vi "Ko.vi"(8 "Model":T3=enum."Gallas", 9 "Thermo and Transport Properties":T1, 10 "SJ Geometry":T2, 11 "omega":dbl=0.001) -> (2 "Ko":dbl=2.000052200153926)   [LabVIEW 2012]
uses:
  Model.ctl
  Utilities/fluid_properties/fluid_properties.ctl
  <vilib>/Analysis/2dsp.llb/Integral Method.ctl
  <vilib>/Analysis/8numeric.llb/1D Numeric Integration.vi
  <vilib>/Analysis/1siggen.llb/Ramp Pattern by Samples.vi
  <vilib>/Analysis/1siggen.llb/Ramp Pattern by Delta.vi
  <vilib>/Analysis/NI_AALBase.lvlib
  <vilib>/Analysis/NI_AALPro.lvlib
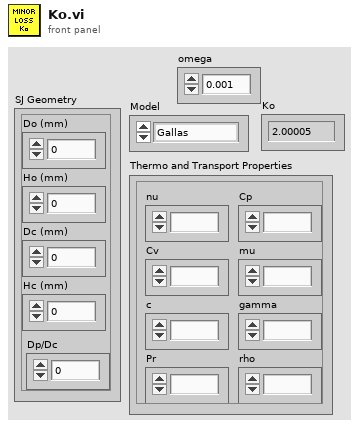
[diagram p1: front panel]
types:
  T1 = typedef "fluid_properties.ctl" = cluster{"nu":dbl, "c":dbl, "Pr":dbl, "Cp":dbl, "Cv":dbl, "gamma":dbl, "mu":dbl, "rho":dbl}
  T2 = cluster{"Do (mm)":dbl, "Ho (mm)":dbl, "Dc (mm)":dbl, "Hc (mm)":dbl, "Dp/Dc":dbl}
  T3 = typedef "Model.ctl" = enum16{"Martin", "Tang", "Gallas", "Persoon"}
  T4 = typedef "NI_AALPro.lvlib/Integral Method.ctl" = i32
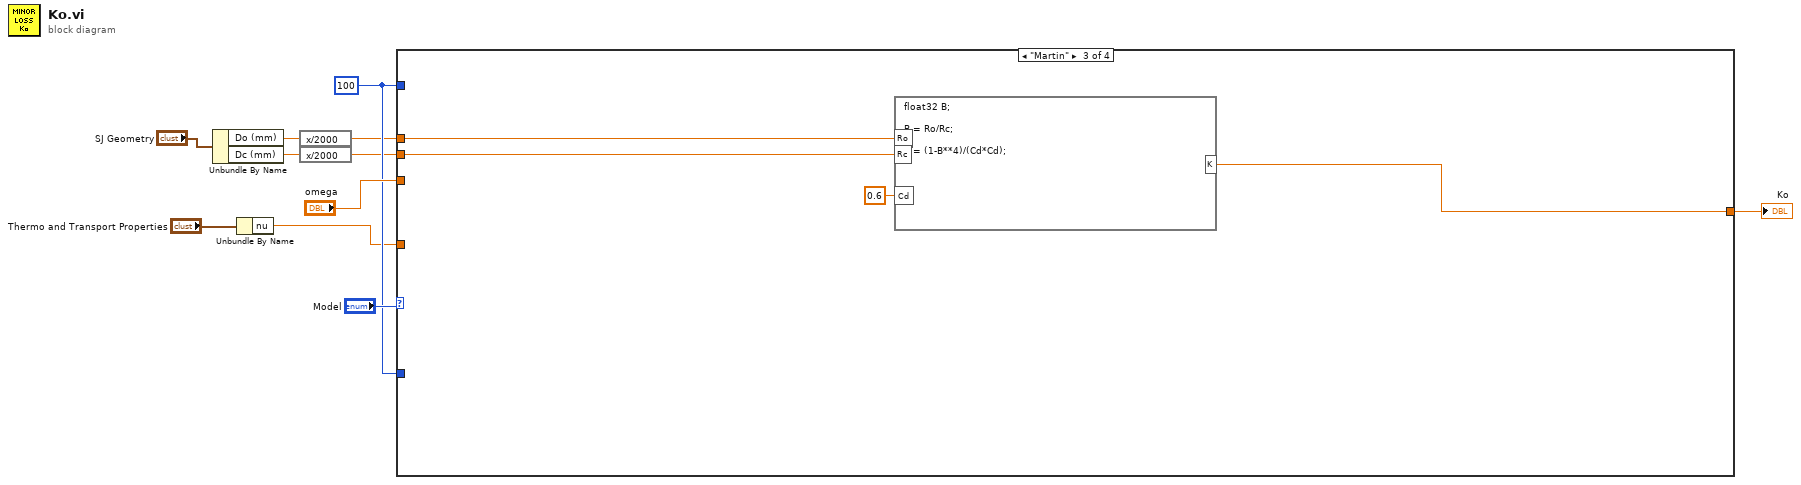
[diagram p0: block diagram]
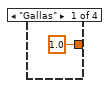
[diagram p2: hidden frame]
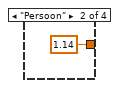
[diagram p3: hidden frame]
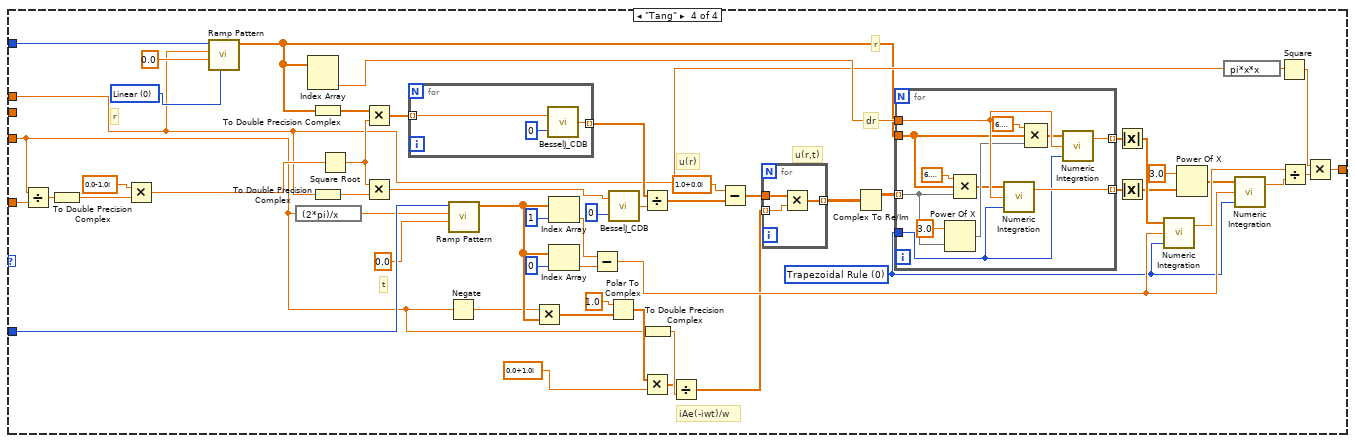
[diagram p4: hidden frame]
diagram:
  w9 = 100 ("n radial pts")
  n1 = Unbundle By Name("SJ Geometry") -> ("Do (mm)"=w7:dbl, "Dc (mm)"=w2:dbl)
  n2 = Unbundle By Name("Thermo and Transport Properties") -> ("nu"=w4:dbl)
  n3 = expression code="x/2000"(w7) -> (w6:dbl)
  n4 = expression code="x/2000"(w2) -> (w1:dbl)
  n5 = case shown="\"Martin\"" "Model" {
    tunnel: [1.0 1.14 w14 w72] -> w3
    tunnel: w4 -> [_ _ _ w57]
    tunnel: w9 -> [_ _ _ w36]
    tunnel: w9 -> [_ _ _ w32]
    tunnel: "omega" -> [_ _ _ w29]
    tunnel: w6 -> [_ _ w17 w27]
    tunnel: w1 -> [_ _ w16 _]
    frame "Gallas" {
    }
    frame "Persoon" {
    }
    frame "Martin" {
      n6 = formula code="float32 B;\n\nB = Ro/Rc;\n\nK = (1-B**4)/(Cd*Cd);"("Ro"=w17, "Rc"=w16, "Cd"=0.6 ("input variable")) -> ("K"=w14:dbl)
    }
    frame "Tang" {
      w23 = T4 0 items=["Trapezoidal Rule", "Simpson's Rule", "Simpson's 3/8 Rule", "Bode Rule"] ("integration method")
      w33 = u16 0 items=["Linear", "Logarithmic"] ("type")
      # "r"
      # "r"
      # "dr"
      # "u(r)"
      # "u(r,t)"
      # "t"
      # "iAe(-iwt)/w"
      n7 = Divide(x=w29, y=w57) -> (x/y=w58:dbl)
      n8 = To Double Precision Complex(1:w58) -> (0:w59:cdb)
      n9 = Multiply(x=cdb 0.0-1.0i, y=w59) -> (x*y=w60:cdb)
      n10 = call-poly <vilib>:"Ramp Pattern.vi"("type"=w33, "start"=0.0, "end"=w27, "samples"=w32) -> ("Ramp Pattern"=w24:dbl[])  [unwired: 6 in, 1 out]
      n11 = expression code="(2*pi)/x"(w29) -> (w28:dbl)
      n12 = Index Array(array=w24) -> (element #2=w31:dbl)  [unwired: 2 in, 1 out]
      n13 = To Double Precision Complex(1:w24) -> (0:w25:cdb[])
      n14 = To Double Precision Complex(1:w27) -> (0:w30:cdb)
      n15 = Square Root(x=w60) -> (sqrt(x)=w62:cdb)
      n16 = Multiply(x=w25, y=w62) -> (x*y=w61:cdb[])
      n17 = Multiply(x=w62, y=w30) -> (x*y=w20:cdb)
      n18 = for {
        tunnel: w61 -> [w75] mode=indexing
        tunnel: [w73] -> w63 mode=indexing
        n19 = call "BesselJ_CDB.vi"("n"=0, "a+bi"=w75) -> ("Jn(a+bi)"=w73:cdb)
      }
      n20 = Negate(x=w29) -> (-x=w43:dbl)
      n21 = call-poly <vilib>:"Ramp Pattern.vi"("start"=0.0, "end"=w28, "samples"=w36) -> ("Ramp Pattern"=w69:dbl[])  [unwired: 7 in, 1 out]
      n22 = Multiply(x=w43, y=w69) -> (x*y=w41:dbl[])
      n23 = Index Array(array=w69, index=1) -> (element=w46:dbl)
      n24 = Index Array(array=w69, index=0) -> (element=w47:dbl)
      n25 = Subtract(x=w46, y=w47) -> (x-y=w54:dbl)
      n26 = Polar To Complex(1:w41, 2:1.0 ("r")) -> (0:w40:cdb[])
      n27 = call "BesselJ_CDB.vi"("n"=0, "a+bi"=w20) -> ("Jn(a+bi)"=w18:cdb)
      n28 = Divide(x=w63, y=w18) -> (x/y=w64:cdb[])
      n29 = Multiply(x=w40, y=cdb 0.0+1.0i) -> (x*y=w38:cdb[])
      n30 = To Double Precision Complex(1:w29) -> (0:w39:cdb)
      n31 = Divide(x=w38, y=w39) -> (x/y=w42:cdb[])
      n32 = Subtract(x=cdb 1.0+0.0i, y=w64) -> (x-y=w67:cdb[])
      n33 = for {
        tunnel: w67 -> [w90]
        tunnel: w42 -> [w89] mode=indexing
        tunnel: [w88] -> w66 mode=indexing
        n34 = Multiply(x=w90, y=w89) -> (x*y=w88:cdb[])
      }
      n35 = Complex To Re/Im(x + iy=w66) -> (x=w68:dbl[][])  [unwired: 1 out]
      n36 = for {
        tunnel: w68 -> [w78] mode=indexing
        tunnel: w31 -> [w85]
        tunnel: [w86] -> w48 mode=indexing
        tunnel: [w84] -> w50 mode=indexing
        tunnel: w24 -> [w80]
        tunnel: w23 -> [w76]
        n37 = Power Of X(1:w78, 2:3.0) -> (0:w82:dbl[])
        n38 = Compound Arithmetic op=MULTIPLY(6.283185307179586, w80, w78) -> (w77:dbl[])
        n39 = call-poly <vilib>:"Numeric Integration.vi"("integration method"=w76, "dt"=w85, "Input Array"=w77) -> ("result"=w84:dbl)  [unwired: 1 out]
        n40 = Compound Arithmetic op=MULTIPLY(6.283185307179586, w80, w82) -> (w81:dbl[])
        n41 = call-poly <vilib>:"Numeric Integration.vi"("integration method"=w76, "dt"=w85, "Input Array"=w81) -> ("result"=w86:dbl)  [unwired: 1 out]
      }
      n42 = Absolute Value(x=w48) -> (abs(x)=w52:dbl[])
      n43 = Absolute Value(x=w50) -> (abs(x)=w51:dbl[])
      n44 = call-poly <vilib>:"Numeric Integration.vi"("integration method"=w23, "dt"=w54, "Input Array"=w52) -> ("result"=w55:dbl)  [unwired: 1 out]
      n45 = Power Of X(1:w51, 2:3.0) -> (0:w53:dbl[])
      n46 = expression code="pi*x*x"(w27) -> (w26:dbl)
      n47 = call-poly <vilib>:"Numeric Integration.vi"("integration method"=w23, "dt"=w54, "Input Array"=w53) -> ("result"=w70:dbl)  [unwired: 1 out]
      n48 = Square(x=w26) -> (x^2=w22:dbl)
      n49 = Divide(x=w55, y=w70) -> (x/y=w71:dbl)
      n50 = Multiply(x=w22, y=w71) -> (x*y=w72:dbl)
    }
  }
  "Ko" <- w3
